vi "64bit-num.vi"(7 "format":bool, 8 "end bit":u64=15, 9 "start bit":u64, 11 "framedata":u64[](array[numeric])) -> (2 "result":u64)   [LabVIEW 2016]
panel:
  out "frameout":u64[](array[numeric])
  out "source":u64
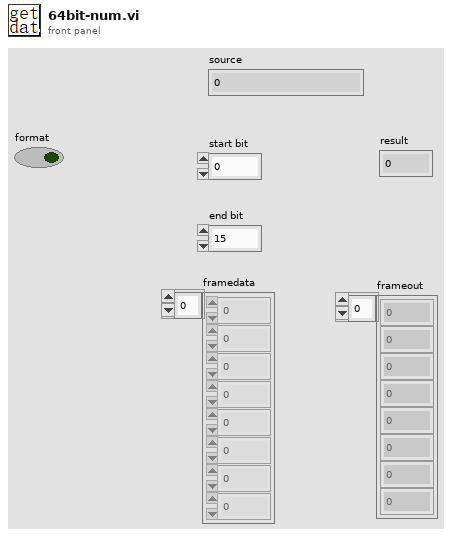
[diagram p1: front panel]
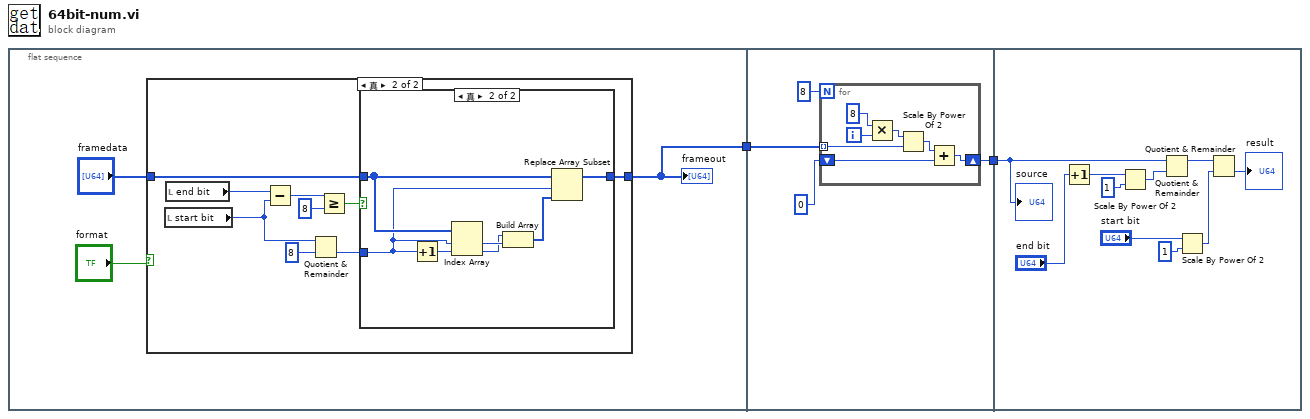
[diagram p0: block diagram]
diagram:
  n1 = flat-sequence {
    tunnel: [w3] -> w1
    tunnel: [w26] -> w2
    tunnel: w1 -> [w24]
    tunnel: w2 -> [w35]
    frame #0 {
      n2 = case shown="真" "format" {
        tunnel: [w6 w8] -> w3
        tunnel: "framedata" -> [w6 w7]
        frame False {
        }
        frame True {
          n3 = local read "start bit"() -> (w12:u64)
          n4 = local read "end bit"() -> (w15:u64)
          n5 = Subtract(x=w15, y=w12) -> (x-y=w14:u64)
          n6 = Quotient & Remainder(x=w12, y=u64 8) -> (floor(x/y)=w10:u64)  [unwired: 1 out]
          n7 = Greater Or Equal?(x=w14, y=u64 8) -> (x >= y?=w9:bool)
          n8 = case shown="真" w9 {
            tunnel: w7 -> [w16 w23]
            tunnel: w10 -> [_ w21]
            tunnel: [w16 w17] -> w8
            frame False {
            }
            frame True {
              n9 = Increment(x=w21) -> (x+1=w22:u64)
              n10 = Index Array(array=w23, index #1=w21, index #2=w22) -> (element #1=w20:u64, element #2=w19:u64)
              n11 = Build Array(w19, w20) -> (w18:u64[])
              n12 = Replace Array Subset(array=w23, new element=w18, index=w21) -> (w17:u64[])
            }
          }
        }
      }
      "frameout" <- w3
    }
    frame #1 {
      n13 = for {
        N: 8 -> [_]
        shift-right: [w29] -> w26
        shift-left: 0 -> [w30]
        tunnel: w24 -> [w28] mode=indexing
        i -> [w31]
        n14 = Multiply(x=8, y=w31) -> (x*y=w33:i32)
        n15 = Scale By Power Of 2(n=w33, x=w28) -> (x*2^n=w32:u64)
        n16 = Add(x=w32, y=w30) -> (x+y=w29:u64)
      }
    }
    frame #2 {
      n17 = Increment(x="end bit") -> (x+1=w37:u64)
      n18 = Scale By Power Of 2(n=w37, x=u64 1) -> (x*2^n=w43:u64)
      n19 = Quotient & Remainder(x=w35, y=w43) -> (x-y*floor(x/y)=w42:u64)  [unwired: 1 out]
      n20 = Scale By Power Of 2(n="start bit", x=u64 1) -> (x*2^n=w40:u64)
      n21 = Quotient & Remainder(x=w42, y=w40) -> (floor(x/y)=→"result":u64)  [unwired: 1 out]
      "source" <- w35
    }
  }
